vi "DI Post Step.vi"(8 "error in (no error)":errorcluster, 9 "DI In":T1, 10 "Socket No":u16=1, 11 "DI in":refnum<class "DI.lvclass">) -> (0 "error out":errorcluster, 1 "DigitalRead":bool[](array[boolean]), 2 "Report Text":string, 3 "DI out":refnum<class "DI.lvclass">, 4 "PhysicalChannel":string[](array[string]))   [LabVIEW 2023, in "HardwareAbstractionLayer_LVOOP.lvlib" / "DI.lvclass"]
uses:
  DI.lvclass
  Control/DI Step Control.ctl
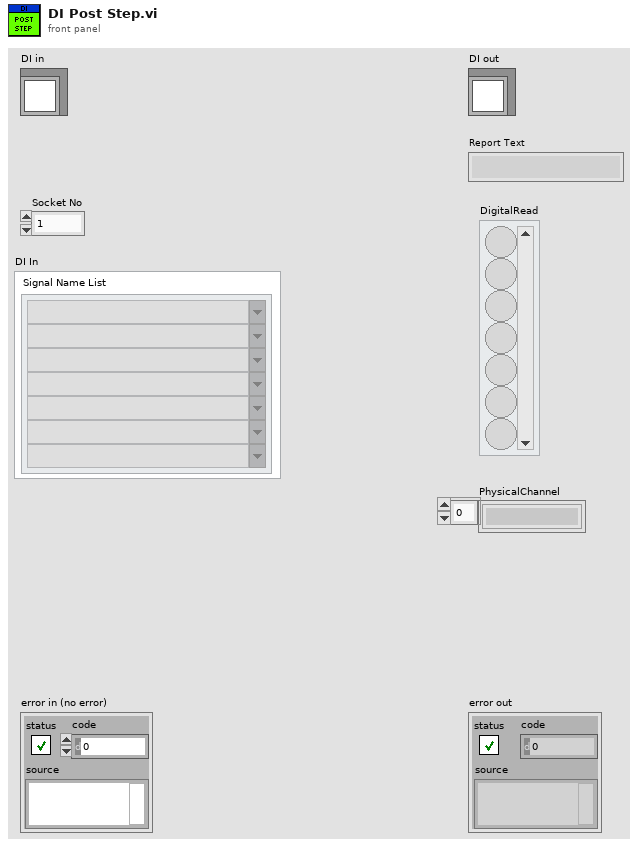
[diagram p1: front panel]
types:
  T1 = typedef "HardwareAbstractionLayer_LVOOP.lvlib/DI.lvclass/DI Step Control.ctl" = cluster{"Signal Name List":string[]}
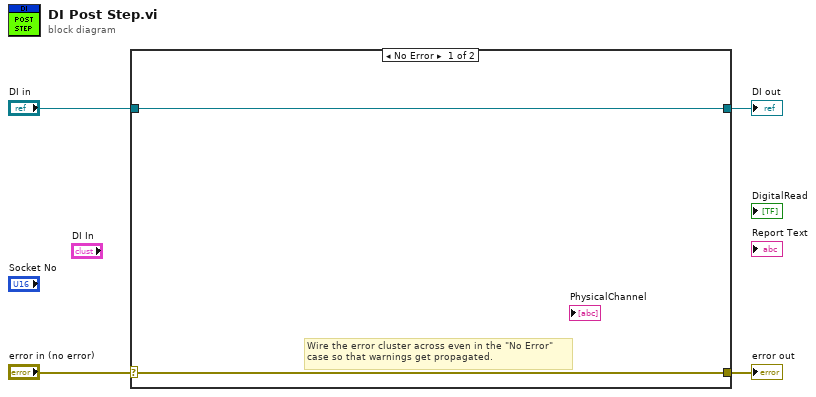
[diagram p0: block diagram]
diagram:
  n1 = case shown="No Error" "error in (no error)" {
    selector: "error in (no error)" -> [w5 w8]
    tunnel: [w5 w8] -> w3
    tunnel: [w6 w7] -> w1
    tunnel: "DI in" -> [w6 w7]
    frame No Error {
      # "Wire the error cluster across even in the \"No Error\"\ncase so that warnings get propagated."
    }
    frame Error {
    }
  }
  "error out" <- w3
  "DI out" <- w1
